vi "test Get and Set Performance.vi"(8 "error in (no error)":errorcluster, 11 "TestCase in":refnum<class "Framework Status Tests.lvclass">) -> (0 "error out":errorcluster, 3 "TestCase out":refnum<class "Framework Status Tests.lvclass">)   [LabVIEW 2017, in "Framework Status Tests.lvclass"]
uses:
  Framework Status Tests.lvclass
  Engine/Classes/Status/Framework Performance.lvclass
  Engine/Classes/Status/Framework Performance.lvclass/Framework Performance.ctl
  Engine/Classes/Status/Framework Status.lvclass/Framework Status.ctl
  <vilib>/addons/_JKI Toolkits/VI Tester/TestCase.llb/TestCase.lvclass
  Engine/Classes/Status/Framework Status.lvclass
  C:/Program Files (x86)/National Instruments/LabVIEW 2017/vi.lib/addons/_JKI Toolkits/VI Tester/TestCase.llb/TestCase.lvclass
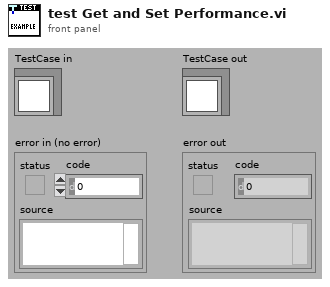
[diagram p1: front panel]
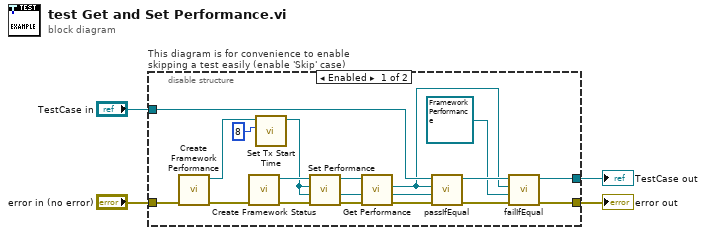
[diagram p0: block diagram]
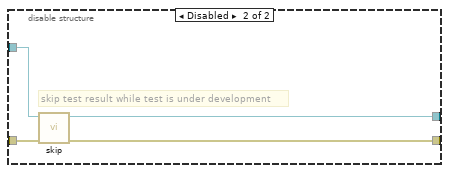
[diagram p2: hidden frame]
diagram:
  n1 = disable-structure "This diagram is for convenience to enable skipping a test easily (enable 'Skip' case)" shown="Enabled" {
    disable-tunnel: "TestCase in" -> [w18 w23]
    disable-tunnel: [w7 w21] -> w1
    disable-tunnel: [w9 w22] -> w3
    disable-tunnel: "error in (no error)" -> [w13 w20]
    frame Enabled {
      n2 = call "Create Framework Performance.vi"("error in (no error)"=w13) -> ("error out"=w12:errorcluster, "Framework Performance"=w15:refnum<class "Framework Performance.lvclass">)  [unwired: 9 in]
      n3 = call "Create Framework Status.vi"("error in (no error)"=w12) -> ("error out"=w11:errorcluster, "Framework Status"=w17:refnum<class "Framework Status.lvclass">)  [unwired: 9 in]
      n4 = call "Set Tx Start Time.vi"("Tx start time"=u32 8, "Framework Performance in"=w15) -> ("Framework Performance out"=w10:refnum<class "Framework Performance.lvclass">)  [unwired: 9 in]
      n5 = call "Set Performance.vi"("Framework Performance"=w10, "Framework Status in"=w17) -> ("Framework Status out"=w16:refnum<class "Framework Status.lvclass">)  [unwired: 9 in]
      n6 = call "Get Performance.vi"("Framework Status in"=w16) -> ("Framework Performance"=w6:refnum<class "Framework Performance.lvclass">)  [unwired: 9 in, 1 out]
      n7 = call-dynamic "passIfEqual.vi"("error in (no error)"=w11, "y"=w10, "x"=w6, "TestCase in"=w18) -> ("error out"=w19:errorcluster, "TestCase out"=w8:refnum<class "Framework Status Tests.lvclass">)  [unwired: 6 in]
      n8 = call-dynamic "failIfEqual.vi"("error in (no error)"=w19, "y"=refnum<class "Framework Performance.lvclass"> refnum ("Framework Performance"), "x"=w6, "TestCase in"=w8) -> ("error out"=w9:errorcluster, "TestCase out"=w7:refnum<class "Framework Status Tests.lvclass">)  [unwired: 6 in]
    }
    frame Disabled {
      # "skip test result while test is under development"
      n9 = call <vilib>:"skip.vi"("error in (no error)"=w20, "TestCase in"=w23) -> ("error out"=w22:errorcluster, "TestCase out"=w21:refnum<class "Framework Status Tests.lvclass">)  [unwired: 8 in]
    }
  }
  "error out" <- w3
  "TestCase out" <- w1
